vi "BRig_Host__Loop_Consumer_RunState__updatePlot.vi"(5 "input_idx":i32[](array[numeric]), 6 "input_DisplayNumber":u16, 7 "input_dataPlot":u16[][](array[numeric]), 11 "input_updatePlot":bool) -> (0 "output_X_min":dbl, 1 "output_X_max":dbl, 2 "output_X_inc":dbl, 3 "XY Graph":cluster{u16[], u16[]}[](graph))   [LabVIEW 2014]
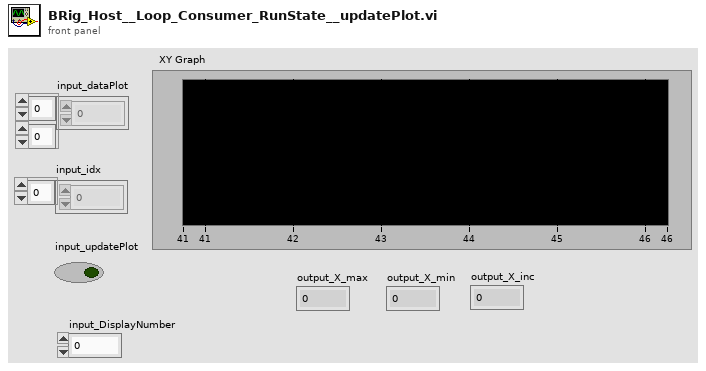
[diagram p1: front panel]
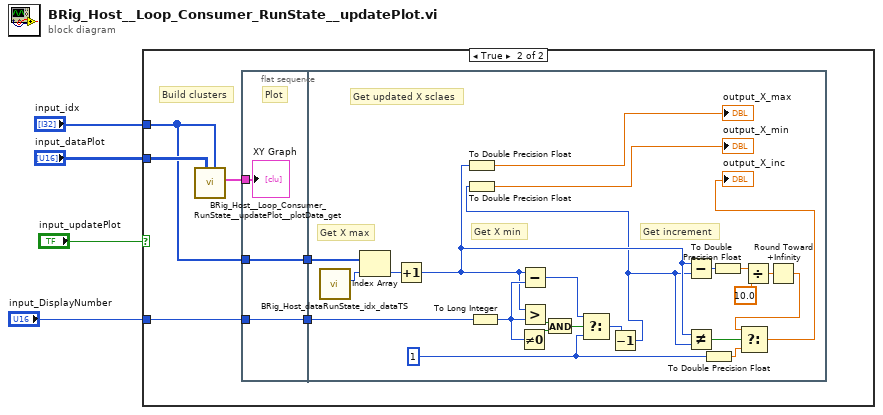
[diagram p0: block diagram]
diagram:
  n1 = case shown="True" "input_updatePlot" {
    tunnel: "input_idx" -> [_ w5]
    tunnel: "input_dataPlot" -> [_ w10]
    tunnel: "input_DisplayNumber" -> [_ w7]
    frame False {
    }
    frame True {
      # "Build clusters"
      n2 = call "BRig_Host__Loop_Consumer_RunState__updatePlot__plotData_get.vi"("input_idx"=w5, "input_dataPlot"=w10) -> ("output_plotData"=w9:cluster{u16[], u16[]}[])  [unwired: 9 in]
      n3 = flat-sequence {
        tunnel: w9 -> [w13]
        tunnel: [w12] -> w8
        tunnel: w7 -> [w12]
        tunnel: [w11] -> w6
        tunnel: w5 -> [w11]
        tunnel: w8 -> [w34]
        tunnel: w6 -> [w36]
        frame #0 {
          # "Plot"
          "XY Graph" <- w13
        }
        frame #1 {
          w22 = 1 ("t")
          # "Get increment"
          # "Get X min"
          # "Get X max"
          # "Get updated X sclaes"
          n4 = call "BRig_Host_dataRunState_idx_dataTS.vi"() -> ("output_idx_dataTS"=w35:i32)  [unwired: 11 in]
          n5 = Index Array(array=w36, index=w35) -> (element=w19:i32)
          n6 = Increment(x=w19) -> (x+1=w18:i32)
          n7 = To Double Precision Float(number=w18) -> (double precision float=→"output_X_max":dbl)
          n8 = To Long Integer(number=w34) -> (32bit integer=w31:i32)
          n9 = Not Equal To 0?(x=w31) -> (x != 0?=w33:bool)
          n10 = Subtract(x=w18, y=w31) -> (x-y=w27:i32)
          n11 = Greater?(x=w18, y=w31) -> (0:w32:bool)
          n12 = And(x=w32, y=w33) -> (x .and. y?=w30:bool)
          n13 = Select(t=w27, s=w30, f=w22) -> (s? t:f=w15:i32)
          n14 = Decrement(x=w15) -> (x-1=w14:i32)
          n15 = To Double Precision Float(number=w14) -> (double precision float=→"output_X_min":dbl)
          n16 = Subtract(x=w18, y=w14) -> (x-y=w29:i32)
          n17 = Not Equal?(x=w18, y=w14) -> (x != y?=w28:bool)
          n18 = To Double Precision Float(number=w22) -> (double precision float=w21:dbl)
          n19 = To Double Precision Float(number=w29) -> (double precision float=w25:dbl)
          n20 = Divide(x=w25, y=10.0) -> (x/y=w24:dbl)
          n21 = Round Toward +Infinity(x=w24) -> (ceil(x): smallest int >= x=w23:dbl)
          n22 = Select(t=w23, s=w28, f=w21) -> (s? t:f=→"output_X_inc":dbl)
        }
      }
    }
  }
